vi "Get Motor Velocity Setpoint.vi"(8 "error in (no error)":errorcluster, 11 "motor communication in":refnum<class "NI_Robotics_Motor Communication.lvclass">) -> (0 "error out":errorcluster, 1 "failed?":bool, 2 "velocity":dbl, 3 "motor communication out":refnum<class "NI_Robotics_Motor Communication.lvclass">)   [LabVIEW 2017, in "NI_Robotics_Motor Communication.lvclass"]
doc: "Returns the angles or angular velocity setpoints from the motor communication session. You must manually select the polymorphic instance to use."
uses:
  <vilib>/robotics/Actuation/Motor Communication/NI_Robotics_Motor Communication.lvclass
  <vilib>/robotics/Actuation/Motor Communication/Motor State Mode.ctl
  <vilib>/robotics/Utilities/Generate Error.vi
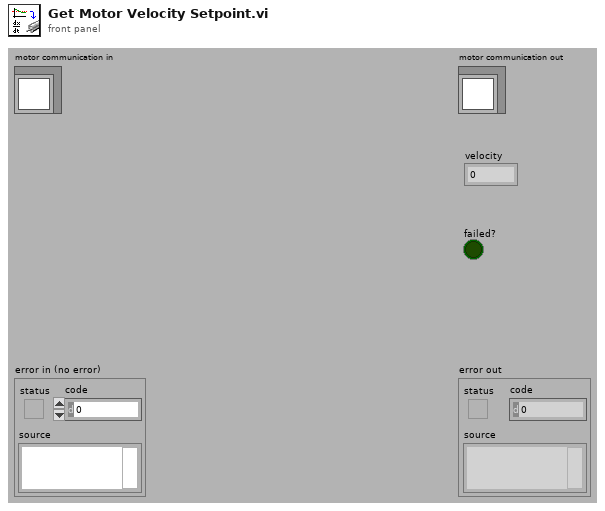
[diagram p1: front panel]
types:
  T1 = typedef "NI_Robotics_Motor Communication.lvclass/Motor State Mode.ctl" = u16
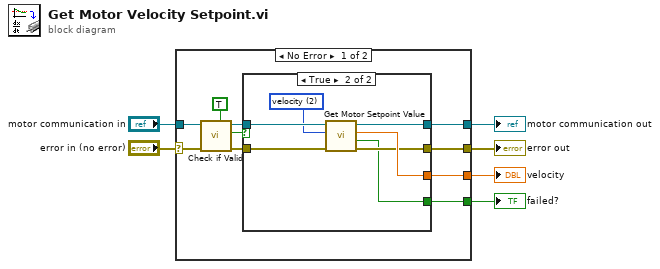
[diagram p0: block diagram]
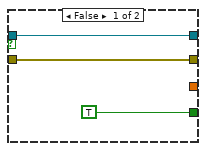
[diagram p2: hidden frame]
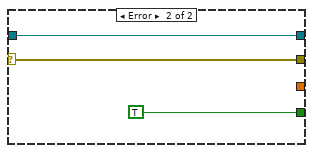
[diagram p3: hidden frame]
diagram:
  n1 = case shown="No Error" "error in (no error)" {
    selector: "error in (no error)" -> [w10 w29]
    tunnel: [w14 w29] -> w5
    tunnel: [w16 w28] -> w3
    tunnel: "motor communication in" -> [w12 w28]
    tunnel: [w15 _] -> w2
    tunnel: [w13 TRUE ("failed")] -> w1
    frame No Error {
      n2 = call <vilib>:"Check if Valid.vi"("produce error if invalid (F)"=TRUE ("generate error if invalid (F)"), "error in (no error)"=w10, "motor communication in"=w12) -> ("error out"=w9:errorcluster, "valid?"=w8:bool, "motor communication out"=w11:refnum<class "NI_Robotics_Motor Communication.lvclass">)  [unwired: 6 in]
      n3 = case shown="True" w8 {
        tunnel: [w19 w26] -> w16
        tunnel: [_ w25] -> w15
        tunnel: [w18 w24] -> w14
        tunnel: [TRUE ("failed") w23] -> w13
        tunnel: w11 -> [w19 w22]
        tunnel: w9 -> [w18 w21]
        frame False {
        }
        frame True {
          w20 = T1 2 items=["undefined", "angle", "velocity"] ("state mode")
          n4 = call-dynamic "Get Motor Setpoint Value.vi"("error in (no error)"=w21, "state mode"=w20, "motor communication in"=w22) -> ("error out"=w24:errorcluster, "failed?"=w23:bool, "value"=w25:dbl, "motor communication out"=w26:refnum<class "NI_Robotics_Motor Communication.lvclass">)  [unwired: 5 in]
        }
      }
    }
    frame Error {
    }
  }
  "error out" <- w5
  "motor communication out" <- w3
  "velocity" <- w2
  "failed?" <- w1
